vi "ConfigurePID.vi"(10 "Right Side":T1) -> ()   [LabVIEW 2017]
uses:
  <vilib>/Rock Robotics/WPI/MotorControl/WPI_MotorControlDeviceRef.ctl
  <vilib>/Rock Robotics/WPI/MotorControl/WPI_MotorControlType.ctl
  <vilib>/Rock Robotics/SystemInterfaces/DIO/FPGA_DIOPWMChannel.ctl
  <vilib>/Rock Robotics/WPI/PWM/WPI_PWMDeadband.ctl
  <vilib>/Rock Robotics/SystemInterfaces/DIO/FPGA_DIOChannel.ctl
  Constants.vi
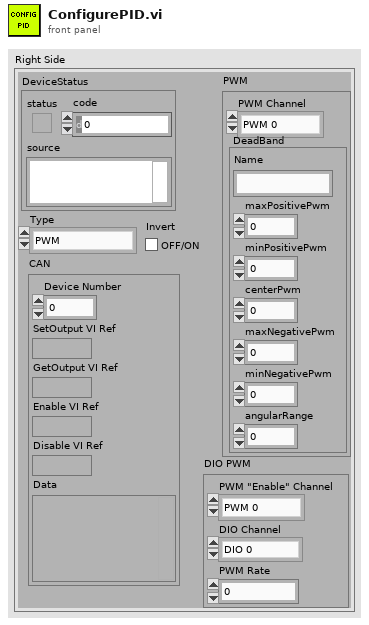
[diagram p1: front panel]
types:
  T1 = typedef "WPI_MotorControlDeviceRef.ctl" = cluster{"DeviceStatus":errorcluster, "Type":T2, "PWM":cluster{"PWM Channel":T3, "DeadBand":T4}, "CAN":cluster{"Device Number":u8, "SetOutput VI Ref":variant, "GetOutput VI Ref":variant, "Enable VI Ref":variant, "Disable VI Ref":variant, "Data":variant}, "Invert":bool, "DIO PWM":cluster{"PWM \"Enable\" Channel":T3, "DIOChannel":T5, "PWM Rate":dbl}}
  T2 = typedef "WPI_MotorControlType.ctl" = enum16{"PWM", "CAN", "DIO PWM"}
  T3 = typedef "FPGA_DIOPWMChannel.ctl" = enum8{"PWM 0", "PWM 1", "PWM 2", "PWM 3", "PWM 4", "PWM 5", "PWM 6", "PWM 7", "PWM 8", "PWM 9", "PWM MXP 0", "PWM MXP 1", "PWM MXP 2", "PWM MXP 3", "PWM MXP 4", "PWM MXP 5", "PWM MXP 6", "PWM MXP 7", "PWM MXP 8", "PWM MXP 9", "Invalid"}
  T4 = typedef "WPI_PWMDeadband.ctl" = cluster{"Name":string, "maxPositivePwm":i32, "minPositivePwm":i32, "centerPwm":i32, "maxNegativePwm":i32, "minNegativePwm":i32, "angularRange":u16}
  T5 = typedef "FPGA_DIOChannel.ctl" = enum8{"DIO 0", "DIO 1", "DIO 2", "DIO 3", "DIO 4", "DIO 5", "DIO 6", "DIO 7", "DIO 8", "DIO 9", "DIO MXP 0", "DIO MXP 1", "DIO MXP 2", "DIO MXP 3", "DIO MXP 4", "DIO MXP 5", "DIO MXP 6", "DIO MXP 7", "DIO MXP 8", "DIO MXP 9", "DIO MXP 10", "DIO MXP 11", "DIO MXP 12", "DIO MXP 13", "DIO MXP 14", "DIO MXP 15", "SPI Port CS1", "SPI Port CS2", "SPI Port CS3", "SPI Port MISO", "SPI Port MOSI", "Invalid"}
  T6 = cluster{"kP":dbl, "kI ":dbl, "kD":dbl, "kF":dbl, "I Zone":dbl, "Peak Out":dbl}
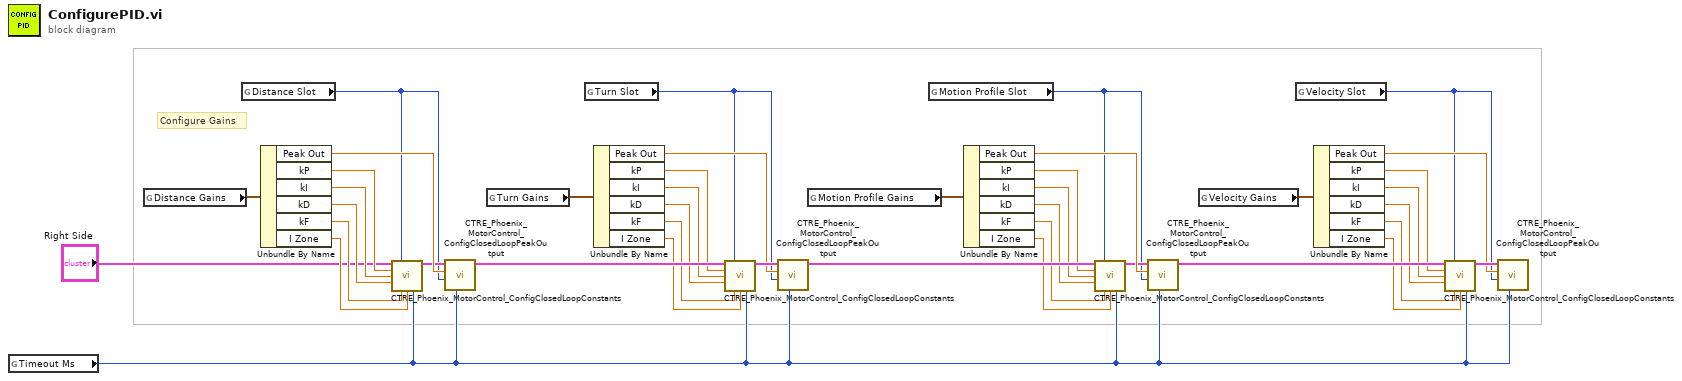
[diagram p0: block diagram]
diagram:
  # "Configure Gains"
  n1 = global read "Constants.vi" "Timeout Ms"() -> (w2:i32)
  n2 = global read "Constants.vi" "Distance Gains"() -> (w7:T6)
  n3 = global read "Constants.vi" "Distance Slot"() -> (w5:i32)
  n4 = Unbundle By Name(w7) -> ("Peak Out"=w14:dbl, "kP"=w8:dbl, "kI"=w9:dbl, "kD"=w10:dbl, "kF"=w11:dbl, "I Zone"=w12:dbl)
  n5 = call <vilib>:"CTRE_Phoenix_MotorControl_ConfigClosedLoopConstants.vi"("PhoenixMotorControlDevRef"="Right Side", "slotIdx"=w5, "P"=w8, "I"=w9, "D"=w10, "F"=w11, "I Zone"=w12, "timeoutMs"=w2) -> ("PhoenixMotorControlDevRef"=w13:T1)  [unwired: 6 in, 1 out]
  n6 = call <vilib>:"CTRE_Phoenix_MotorControl_ConfigClosedLoopPeakOutput.vi"("timoutMs"=w2, "slotIdx"=w5, "peakOutput"=w14, "PhoenixMotorControlDevRef"=w13) -> ("PhoenixMotorControlDevRef"=w39:T1)  [unwired: 6 in, 1 out]
  n7 = global read "Constants.vi" "Turn Gains"() -> (w22:T6)
  n8 = global read "Constants.vi" "Turn Slot"() -> (w4:i32)
  n9 = Unbundle By Name(w22) -> ("Peak Out"=w15:dbl, "kP"=w21:dbl, "kI"=w20:dbl, "kD"=w19:dbl, "kF"=w18:dbl, "I Zone"=w17:dbl)
  n10 = call <vilib>:"CTRE_Phoenix_MotorControl_ConfigClosedLoopConstants.vi"("PhoenixMotorControlDevRef"=w39, "slotIdx"=w4, "P"=w21, "I"=w20, "D"=w19, "F"=w18, "I Zone"=w17, "timeoutMs"=w2) -> ("PhoenixMotorControlDevRef"=w16:T1)  [unwired: 6 in, 1 out]
  n11 = call <vilib>:"CTRE_Phoenix_MotorControl_ConfigClosedLoopPeakOutput.vi"("timoutMs"=w2, "slotIdx"=w4, "peakOutput"=w15, "PhoenixMotorControlDevRef"=w16) -> ("PhoenixMotorControlDevRef"=w40:T1)  [unwired: 6 in, 1 out]
  n12 = global read "Constants.vi" "Motion Profile Gains"() -> (w23:T6)
  n13 = global read "Constants.vi" "Motion Profile Slot"() -> (w6:i32)
  n14 = Unbundle By Name(w23) -> ("Peak Out"=w30:dbl, "kP"=w24:dbl, "kI"=w25:dbl, "kD"=w26:dbl, "kF"=w27:dbl, "I Zone"=w28:dbl)
  n15 = call <vilib>:"CTRE_Phoenix_MotorControl_ConfigClosedLoopConstants.vi"("PhoenixMotorControlDevRef"=w40, "slotIdx"=w6, "P"=w24, "I"=w25, "D"=w26, "F"=w27, "I Zone"=w28, "timeoutMs"=w2) -> ("PhoenixMotorControlDevRef"=w29:T1)  [unwired: 6 in, 1 out]
  n16 = call <vilib>:"CTRE_Phoenix_MotorControl_ConfigClosedLoopPeakOutput.vi"("timoutMs"=w2, "slotIdx"=w6, "peakOutput"=w30, "PhoenixMotorControlDevRef"=w29) -> ("PhoenixMotorControlDevRef"=w41:T1)  [unwired: 6 in, 1 out]
  n17 = global read "Constants.vi" "Velocity Gains"() -> (w38:T6)
  n18 = global read "Constants.vi" "Velocity Slot"() -> (w3:i32)
  n19 = Unbundle By Name(w38) -> ("Peak Out"=w31:dbl, "kP"=w37:dbl, "kI"=w36:dbl, "kD"=w35:dbl, "kF"=w34:dbl, "I Zone"=w33:dbl)
  n20 = call <vilib>:"CTRE_Phoenix_MotorControl_ConfigClosedLoopConstants.vi"("PhoenixMotorControlDevRef"=w41, "slotIdx"=w3, "P"=w37, "I"=w36, "D"=w35, "F"=w34, "I Zone"=w33, "timeoutMs"=w2) -> ("PhoenixMotorControlDevRef"=w32:T1)  [unwired: 6 in, 1 out]
  n21 = call <vilib>:"CTRE_Phoenix_MotorControl_ConfigClosedLoopPeakOutput.vi"("timoutMs"=w2, "slotIdx"=w3, "peakOutput"=w31, "PhoenixMotorControlDevRef"=w32) -> ()  [unwired: 6 in, 2 out]
